vi "Write Laser Enable.vi"(8 "error in (no error)":errorcluster, 10 "Laser Enable":bool[](array[boolean]), 11 "Set f0 MSG in":refnum<class "Set Las Enable MSG.lvclass">) -> (0 "error out":errorcluster, 3 "Set f0 MSG out":refnum<class "Set Las Enable MSG.lvclass">)   [LabVIEW 2014, in "ePAS Library.lvlib" / "Set Las Enable MSG.lvclass"]
uses:
  Set Las Enable MSG.lvclass
  Set Las Enable MSG.lvclass/Set Las Enable MSG.ctl
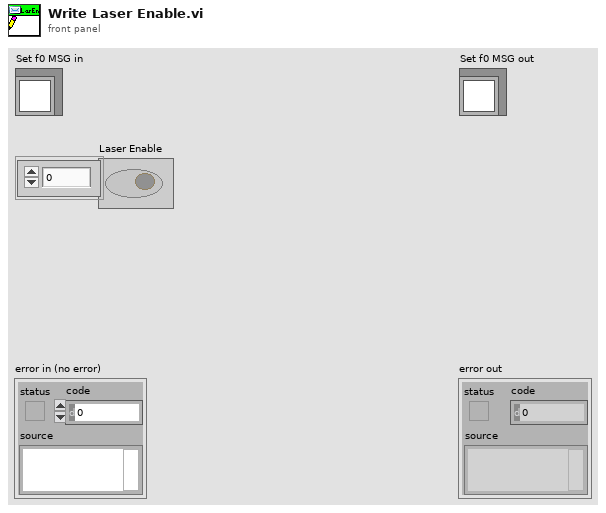
[diagram p1: front panel]
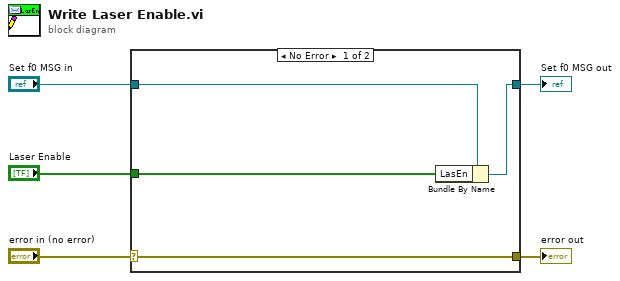
[diagram p0: block diagram]
diagram:
  n1 = case shown="No Error" "error in (no error)" {
    selector: "error in (no error)" -> [w9 w10]
    tunnel: [w9 w10] -> w4
    tunnel: [w7 w11] -> w2
    tunnel: "Set f0 MSG in" -> [w8 w11]
    tunnel: "Laser Enable" -> [w6 _]
    frame No Error {
      n2 = Bundle By Name(cluster=w8, "LasEn"=w6) -> (w7:refnum<class "Set Las Enable MSG.lvclass">)
    }
    frame Error {
    }
  }
  "error out" <- w4
  "Set f0 MSG out" <- w2
